vi "Add Channel.vi"(8 "error in (no error)":errorcluster, 9 "Index":i32, 10 "Name":string, 11 "SignalManager in":refnum<class "SignalManager.lvclass">) -> (0 "error out":errorcluster, 3 "SignalManager out":refnum<class "SignalManager.lvclass">)   [LabVIEW 2015, in "SignalManager.lvclass"]
uses:
  SignalManager.lvclass
  SignalManager.lvclass/SignalManager.ctl
  Channel/Channel.lvclass
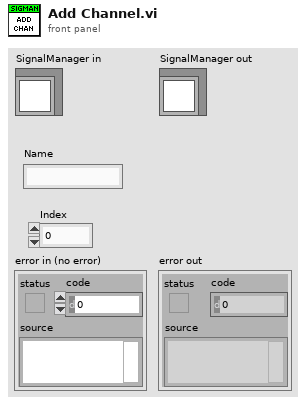
[diagram p1: front panel]
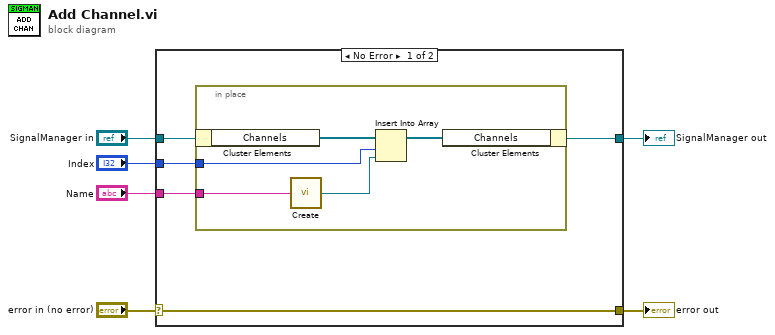
[diagram p0: block diagram]
diagram:
  n1 = case shown="No Error" "error in (no error)" {
    selector: "error in (no error)" -> [w11 w18]
    tunnel: [w11 w18] -> w5
    tunnel: [w9 w17] -> w3
    tunnel: "SignalManager in" -> [w10 w17]
    tunnel: "Index" -> [w8 _]
    tunnel: "Name" -> [w7 _]
    frame No Error {
      n2 = in-place {
        in-place-border: w8 -> [w14]
        in-place-border: w7 -> [w12]
        n3 = in-place-cluster #1(w10) -> ("Channels"=w16:refnum<class "Channel.lvclass">[])
        n4 = call "Create.vi"("Name"=w12) -> ("Channel"=w13:refnum<class "Channel.lvclass">)  [unwired: 14 in]
        n5 = Insert Into Array(array=w16, index=w14, new element=w13) -> (w15:refnum<class "Channel.lvclass">[])
        n6 = in-place-cluster #1("Channels"=w15) -> (w9:refnum<class "SignalManager.lvclass">)
      }
    }
    frame Error {
    }
  }
  "error out" <- w5
  "SignalManager out" <- w3
